vi "TL_erase_all_tasks_TDMS.vi"(2 "error in":errorcluster) -> (0 "error out":errorcluster)   [LabVIEW 2015]
uses:
  GLOBAL/Global_MAIN.vi
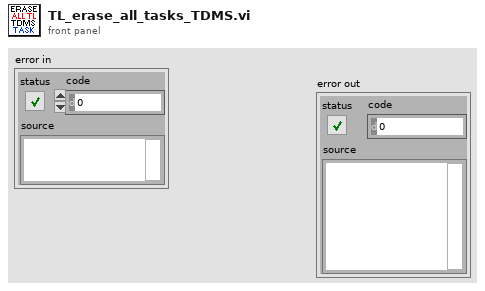
[diagram p1: front panel]
types:
  T1 = enum16{"open", "open or create", "create or replace", "create", "open (read-only)"}
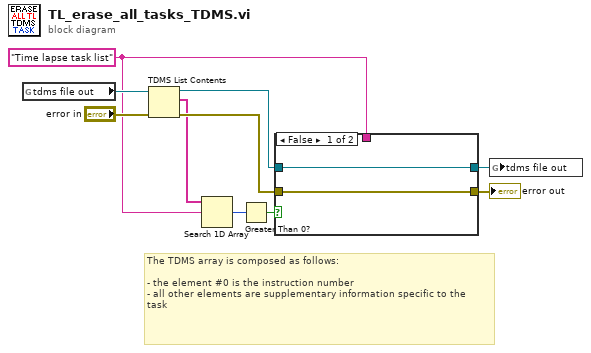
[diagram p0: block diagram]
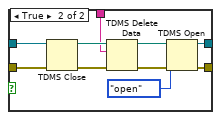
[diagram p2: hidden frame]
diagram:
  w1 = "Time lapse task list" ("group name in (Untitled)")
  # "The TDMS array is composed as follows:\n\n- the element #0 is the instruction number\n- all other elements are supplementary information specific to the\ntask"
  n1 = global read "Global_MAIN.vi" "tdms file out"() -> (w6:refnum<k34>)
  n2 = TDMS List Contents(4:"error in", 7:w6) -> (0:w9:errorcluster, 2:w3:string[], 3:w10:refnum<k34>)  [unwired: 1 in, 1 out]
  n3 = Search 1D Array(1D array=w3, element=w1) -> (index of element=w2:i32)  [unwired: 1 in]
  n4 = Greater Than 0?(x=w2) -> (x > 0?=w5:bool)
  n5 = case shown="False" w5 {
    tunnel: [w12 w19] -> w4
    tunnel: [w11 w18] -> w8
    tunnel: w10 -> [w12 w15]
    tunnel: w9 -> [w11 w14]
    tunnel: w1 -> [_ w13]
    frame False {
    }
    frame True {
      n6 = TDMS Close(8:w14, 11:w15) -> (0:w16:errorcluster, 3:w17:path)
      n7 = TDMS Delete Data(8:w16, 10:w13, 11:w17) -> (0:w21:errorcluster, 3:w22:path)  [unwired: 4 in]
      n8 = TDMS Open(8:w21, 10:T1."open" ("operation (0:open)"), 11:w22) -> (0:w18:errorcluster, 3:w19:refnum<k34>)  [unwired: 4 in]
    }
  }
  "error out" <- w8
  n9 = global write "Global_MAIN.vi" "tdms file out"(w4) -> ()
